vi "Write Data To User File.vi"(8 "error in":errorcluster, 9 "Data":string[][](array[string]), 11 "File path":path) -> (0 "error out":errorcluster)   [LabVIEW 2017]
uses:
  General/Config.llb/_WriteConfiguration(String).vi
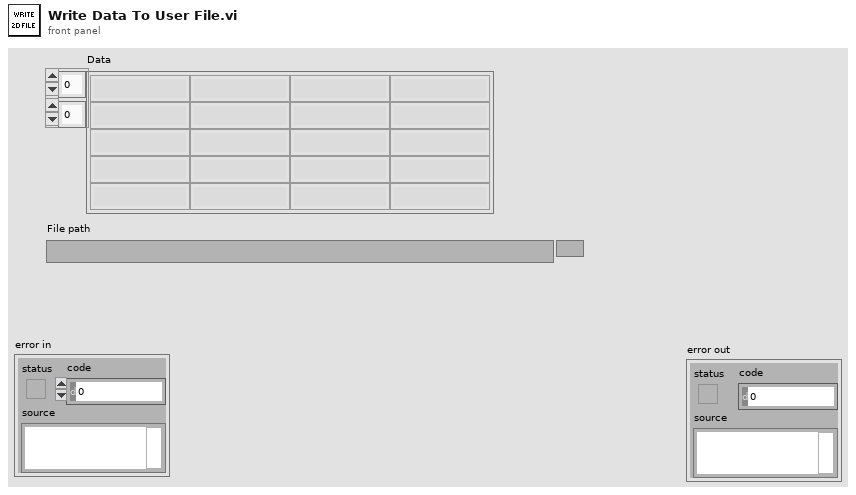
[diagram p1: front panel]
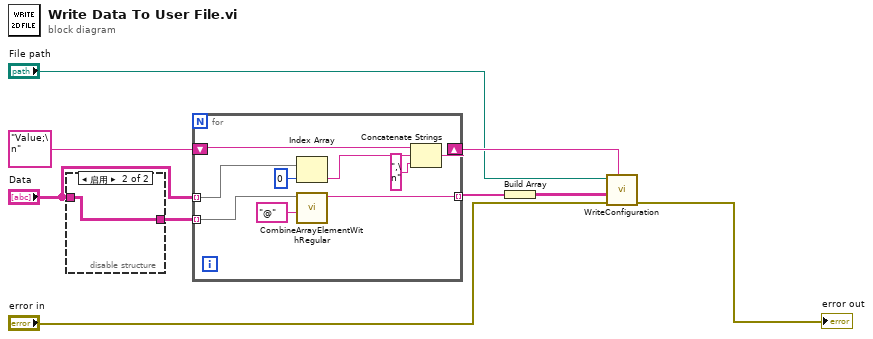
[diagram p0: block diagram]
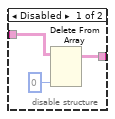
[diagram p2: hidden frame]
diagram:
  n1 = disable-structure shown="启用" {
    disable-tunnel: "Data" -> [w12 w13]
    disable-tunnel: [w10 w13] -> w1
    frame Disabled {
      n2 = Delete From Array(array=w12, index (col)=0 ("禁用的索引 (列)")) -> (array with subset deleted=w10:string[][])  [unwired: 2 in, 1 out]
    }
    frame Enabled {
    }
  }
  n3 = for {
    tunnel: "Data" -> [w14] mode=indexing
    tunnel: [w21] -> w6 mode=indexing
    shift-right: [w17] -> w8
    shift-left: "Value;\n" ("section&key") -> [w19]
    tunnel: w1 -> [w15] mode=indexing
    n4 = Index Array(array=w14, index=0 ("索引")) -> (element=w18:string)
    n5 = call "CombineArrayElementWithRegular.vi"("regular expression"="@", "Array in"=w15) -> ("String out"=w21:string)  [unwired: 9 in]
    n6 = Concatenate Strings(w19, w18, ",\n" ("字符串")) -> (w17:string)
  }
  n7 = Build Array(w6) -> (w5:string[][])
  n8 = call-poly "WriteConfiguration.vi"("section&key"=w8, "error in"="error in", "value"=w5, "configuration file path"="File path") -> ("error out"=→"error out":errorcluster)  [unwired: 4 in, 1 out]
